vi "Example msgQ_handler.vi"(7 "MsgQ enum":T1, 8 "error in (no error)":errorcluster, 9 "Message Send Parameters":variant, 10 "Message Send String":string, 11 "Mode":T2) -> (0 "error out":errorcluster, 1 "Message Received Parameters":variant, 2 "Message Received String":string, 5 "Message Recieved?":bool)   [LabVIEW 2013]
doc: "Create from template a message handler for interloop operations. \n1. Open and sasve a copy in your application.\n2. Replace the enum with a typdef enum list of queue names.\n\nModes:\na. Intialize mode to initialize queues on first call.\nb. Kill mode to destroy all queues at end of use.\nc. broadcast to send a message to all queues\nd. send to sent to a specified loop\ne. read -reads next message in specified queue"
uses:
  Message que instance modes enum.ctl
  Example msgQ names enums.ctl
  Message cluster.ctl
  Message queue handler mode enums.ctl
  Interloop MessageQ.lvlib
  <vilib>/Utility/VariantDataType/VariantType.lvlib
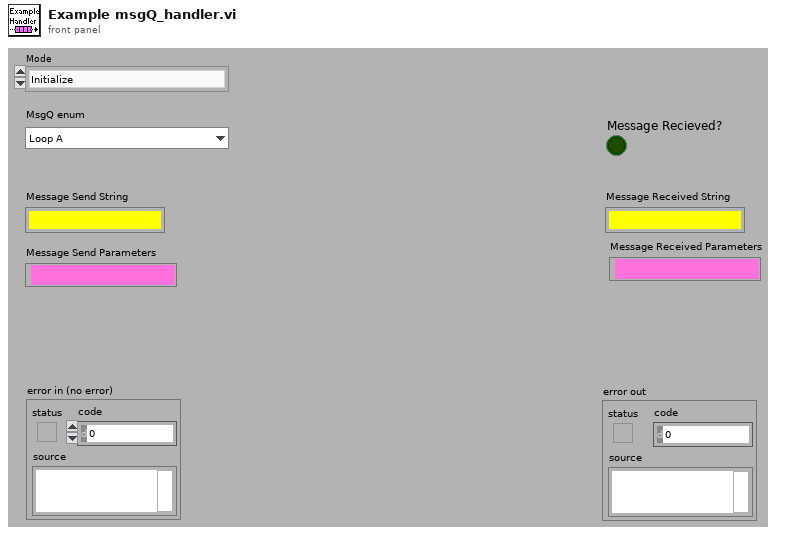
[diagram p1: front panel]
types:
  T1 = typedef "Example msgQ names enums.ctl" = enum16{"Loop A", "Loop B", "Loop C"}
  T2 = typedef "Interloop MessageQ.lvlib/Message que instance modes enum.ctl" = enum16{"Initialize", "Broadcast Message", "Send Message", "Read Message", "Kill"}
  T3 = typedef "Interloop MessageQ.lvlib/Message cluster.ctl" = cluster{"Message String":string, "Data":variant}
  T4 = typedef "Interloop MessageQ.lvlib/Message queue handler mode enums.ctl" = enum16{"Initialize", "Create MsgQ", "Destroy MsgQ", "Send Message", "Broadcast Message", "Read Message", "Close"}
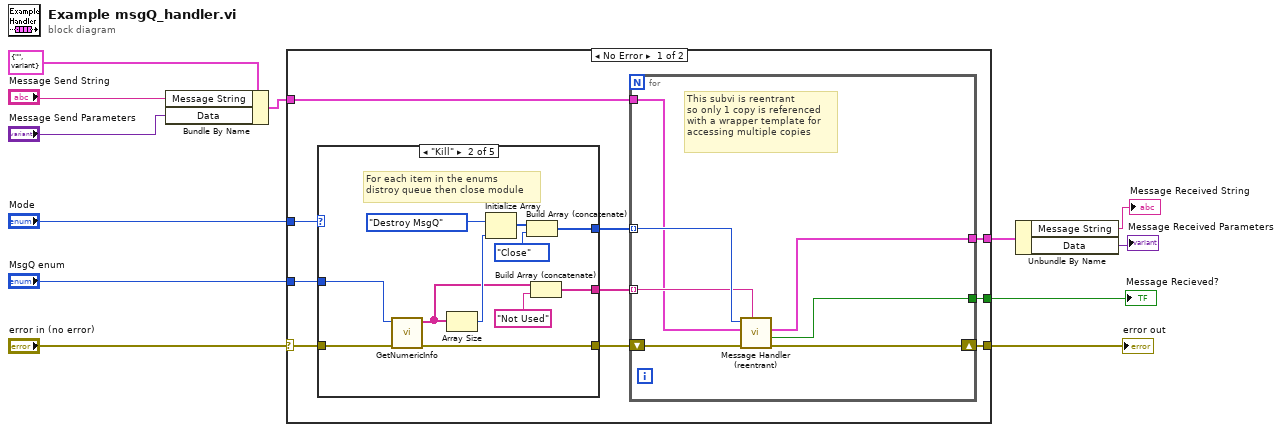
[diagram p0: block diagram]
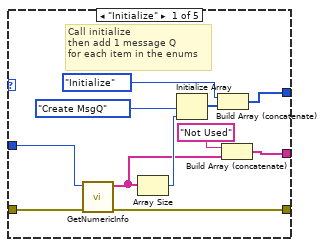
[diagram p2: hidden frame]
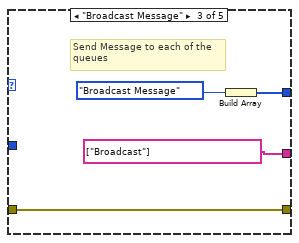
[diagram p3: hidden frame]
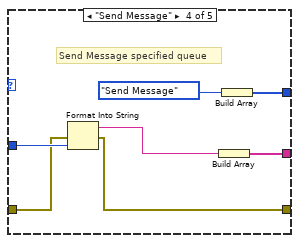
[diagram p4: hidden frame]
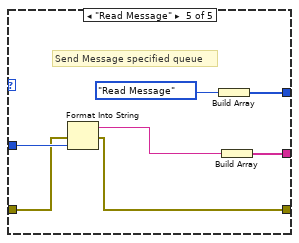
[diagram p5: hidden frame]
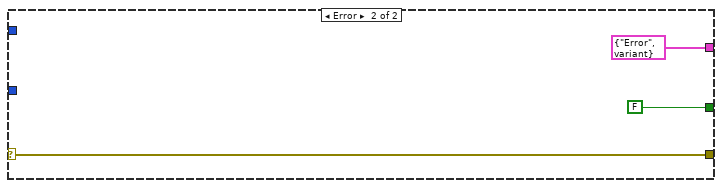
[diagram p6: hidden frame]
diagram:
  n1 = Bundle By Name(cluster=T3 {"Message String"="", "Data"=variant} ("Message to send"), "Message String"="Message Send String", "Data"="Message Send Parameters") -> (w2:T3)
  n2 = case shown="No Error" "error in (no error)" {
    selector: "error in (no error)" -> [w20 w72]
    tunnel: [w22 w72] -> w10
    tunnel: "MsgQ enum" -> [w21 _]
    tunnel: "Mode" -> [w19 _]
    tunnel: [w17 T3 {"Message String"="Error", "Data"=variant} ("Message recieved")] -> w7
    tunnel: [w16 FALSE ("Message Recieved?")] -> w8
    tunnel: w2 -> [w13 _]
    frame No Error {
      n3 = case shown="\"Kill\"" w19 {
        tunnel: w21 -> [w33 w44 _ w53 w60]
        tunnel: w20 -> [w32 w43 w46 w49 w56]
        tunnel: [w31 w42 w46 w50 w57] -> w18
        tunnel: [w26 w38 w47 w54 w61] -> w15
        tunnel: [w23 w36 string[] ["Broadcast"] w51 w58] -> w14
        frame "Initialize" {
          # "Call initialize\nthen add 1 message Q\nfor each item in the enums"
          n4 = call <vilib>:"GetNumericInfo.vi"("error in (no error)"=w32, "Variant"=w33) -> ("error out"=w31:errorcluster, "EnumNames"=w25:string[])  [unwired: 8 out]
          n5 = Array Size(array=w25) -> (size(s)=w28:i32)
          n6 = Initialize Array(Message_queue_handler_mode_enums."Create MsgQ" ("Mode"), w28) -> (w29:T4[])
          n7 = Build Array (concatenate)(Message_queue_handler_mode_enums."Initialize" ("Mode"), w29) -> (w26:T4[])
          n8 = Build Array (concatenate)("Not Used" ("String"), w25) -> (w23:string[])
        }
        frame "Kill" {
          # "For each item in the enums\ndistroy queue then close module"
          n9 = call <vilib>:"GetNumericInfo.vi"("error in (no error)"=w43, "Variant"=w44) -> ("error out"=w42:errorcluster, "EnumNames"=w37:string[])  [unwired: 8 out]
          n10 = Array Size(array=w37) -> (size(s)=w39:i32)
          n11 = Initialize Array(Message_queue_handler_mode_enums."Destroy MsgQ" ("Mode"), w39) -> (w40:T4[])
          n12 = Build Array (concatenate)(w40, Message_queue_handler_mode_enums."Close" ("Mode")) -> (w38:T4[])
          n13 = Build Array (concatenate)(w37, "Not Used" ("String")) -> (w36:string[])
        }
        frame "Broadcast Message" {
          # "Send Message to each of the\nqueues"
          n14 = Build Array(Message_queue_handler_mode_enums."Broadcast Message" ("Mode")) -> (w47:T4[])
        }
        frame "Send Message" {
          # "Send Message specified queue"
          n15 = Format Into String(error in=w49, w53) -> (resulting string=w52:string, error out=w50:errorcluster)  [unwired: 2 in]
          n16 = Build Array(w52) -> (w51:string[])
          n17 = Build Array(Message_queue_handler_mode_enums."Send Message" ("Mode")) -> (w54:T4[])
        }
        frame "Read Message" {
          # "Send Message specified queue"
          n18 = Format Into String(error in=w56, w60) -> (resulting string=w59:string, error out=w57:errorcluster)  [unwired: 2 in]
          n19 = Build Array(Message_queue_handler_mode_enums."Read Message" ("Mode")) -> (w61:T4[])
          n20 = Build Array(w59) -> (w58:string[])
        }
      }
      n21 = for {
        shift-right: [w68] -> w22
        shift-left: w18 -> [w69]
        tunnel: [w67] -> w17
        tunnel: [w66] -> w16
        tunnel: w15 -> [w65] mode=indexing
        tunnel: w14 -> [w64] mode=indexing
        tunnel: w13 -> [w63]
        # "This subvi is reentrant\nso only 1 copy is referenced\nwith a wrapper template for \naccessing multiple copies"
        n22 = call "Message Handler (reentrant).vi"("MsgQ Name"=w64, "error in (no error)"=w69, "Message to send"=w63, "Mode"=w65) -> ("error out"=w68:errorcluster, "Message Recieved?"=w66:bool, "Message recieved"=w67:T3)  [unwired: 5 out]
      }
    }
    frame Error {
    }
  }
  "error out" <- w10
  "Message Recieved?" <- w8
  n23 = Unbundle By Name(w7) -> ("Message String"=→"Message Received String":string, "Data"=→"Message Received Parameters":variant)
